vi "Add Unconfigured NICs.vi"(7 "ifconfig":string="# This file describes the network interfaces available on your system\n# and how to activate them. For more information, see interfaces(5).\n\n# The loopback network interface\nauto lo\niface lo inet loopback\n\n# The primary network interface\n#auto eth0\n#iface eth0 inet dhcp\n# Example to keep MAC address between reboots\n#hwaddress ether DE:AD:BE:EF:CA:FE\n\n# The secondary network interface\n#auto eth1\n#iface eth1 inet dhcp\n\n# WiFi Example\n#auto wlan0\n#iface wlan0 inet dhcp\n#    wpa-ssid \"essid\"\n#    wpa-psk  \"password\"\n\n# Ethernet/RNDIS gadget (g_ether)\n# Used by: /opt/scripts/boot/autoconfigure_usb0.sh\niface usb0 inet static\n    address 192.168.7.2\n    netmask 255.255.255.252\n    network 192.168.7.0\n    gateway 192.168.7.1e", 8 "Error In":errorcluster, 10 "All NIC Names":string[](array[string]), 11 "NIC Configs":T1[](array[typedef])) -> (0 "Error Out":errorcluster, 3 "NIC Configs":T1[](array[typedef]))   [LabVIEW 2020, in "LMH-LINX.lvlib"]
uses:
  LMH-LINX.lvlib
  NIC Info.ctl
  NIC Mode.ctl
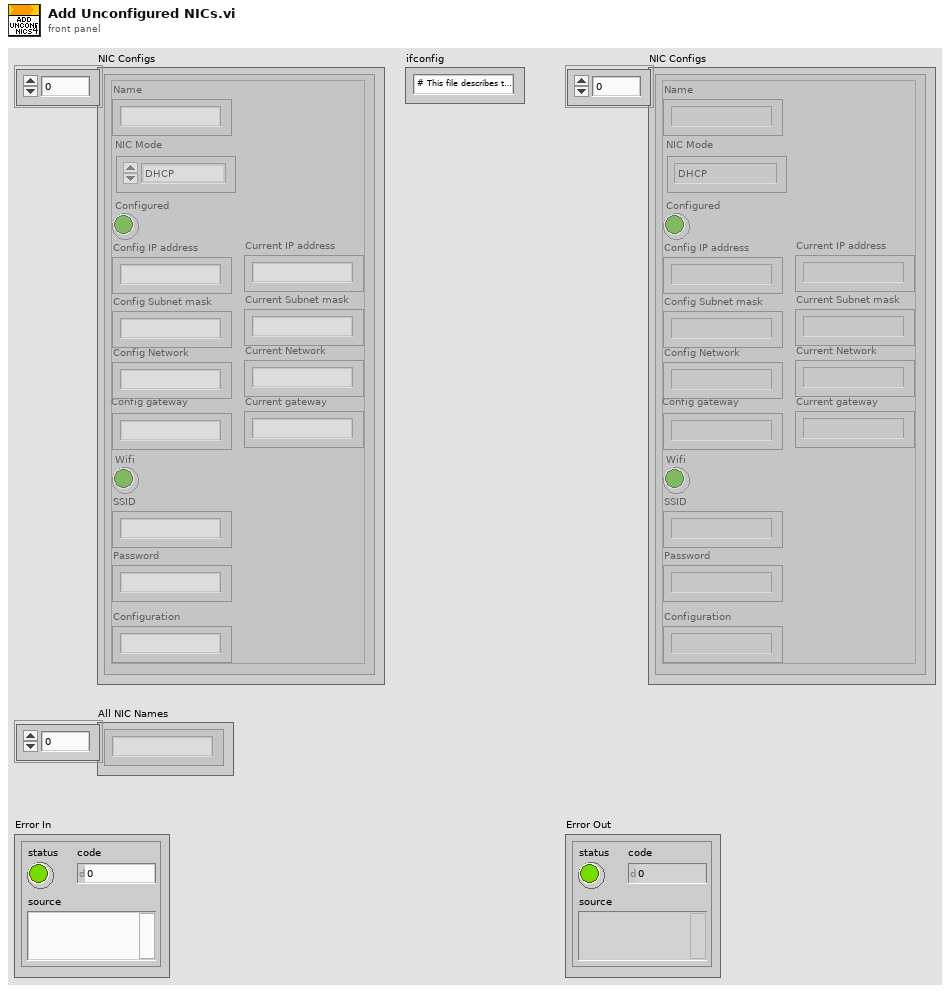
[diagram p1: front panel]
types:
  T1 = typedef "LMH-LINX.lvlib/NIC Info.ctl" = cluster{"Name":string, "NIC Mode":T2, "Configured":bool, "Config IP address":string, "Config Subnet mask":string, "Config Network":string, "Config gateway":string, "Wifi":bool, "SSID":string, "Password":string, "Configuration":string, "Current IP address":string, "Current Subnet mask":string, "Current gateway":string, "Current Network":string}
  T2 = typedef "LMH-LINX.lvlib/NIC Mode.ctl" = enum16{"DHCP", "Static", "Loopback"}
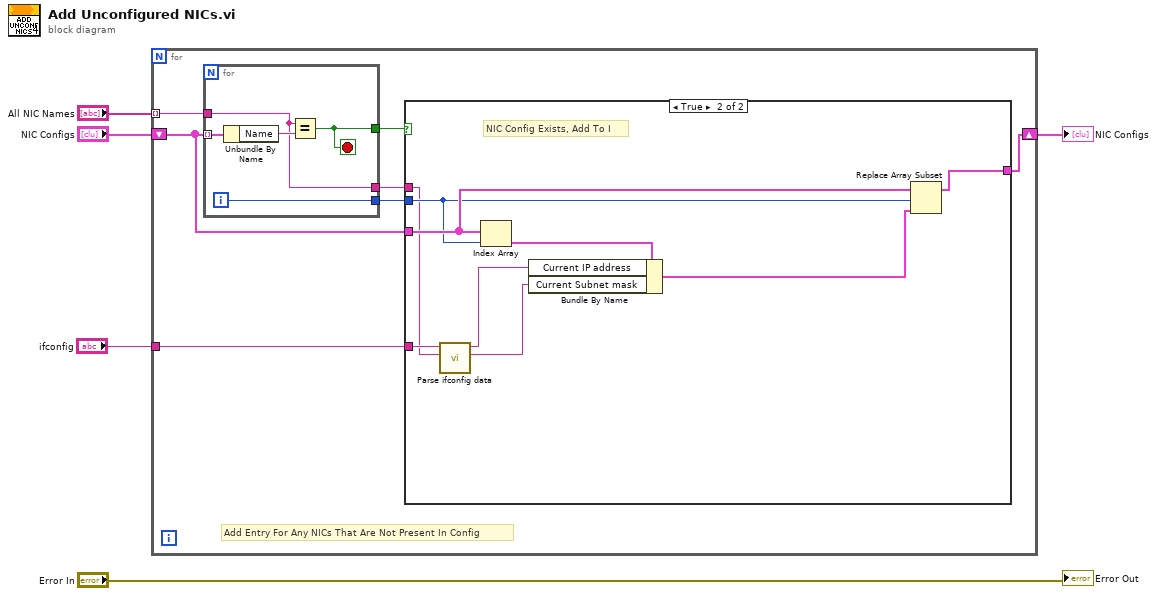
[diagram p0: block diagram]
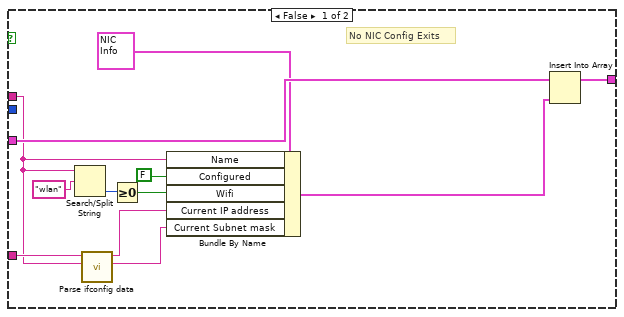
[diagram p2: hidden frame]
diagram:
  n1 = for {
    tunnel: "All NIC Names" -> [w7] mode=indexing
    shift-right: [w11] -> w5
    shift-left: "NIC Configs" -> [w9]
    tunnel: "ifconfig" -> [w8]
    # "Add Entry For Any NICs That Are Not Present In Config"
    n2 = for {
      tunnel: w9 -> [w36] mode=indexing
      tunnel: w7 -> [w35]
      tunnel: [w37] -> w12
      tunnel: [w35] -> w10
      tunnel: [w34] -> w6
      i -> [w34]
      stop <- w37 stop-if-true
      n3 = Unbundle By Name(w36) -> ("Name"=w38:string)
      n4 = Equal?(x=w35, y=w38) -> (x = y?=w37:bool)
    }
    n5 = case shown="True" w12 {
      tunnel: w9 -> [w24 w33]
      tunnel: [w23 w30] -> w11
      tunnel: w10 -> [w15 w25]
      tunnel: w8 -> [w19 w28]
      tunnel: w6 -> [_ w29]
      frame False {
        # "No NIC Config Exits"
        n6 = Search/Split String(string=w15, search string/char (-)="wlan") -> (offset of match=w18:i32)  [unwired: 1 in, 2 out]
        n7 = call "Parse ifconfig data.vi"("NIC Name"=w15, "ifconfig"=w19) -> ("Subnet mask"=w13:string, "IP Address"=w14:string)  [unwired: 8 in]
        n8 = Greater Or Equal To 0?(x=w18) -> (x >= 0?=w16:bool)
        n9 = Bundle By Name(cluster=T1 {"Name"="", "NIC Mode"=enum."DHCP", "Configured"=FALSE, "Config IP address"="", "Config Subnet mask"="", "Config Network"="", "Config gateway"="", "Wifi"=FALSE, "SSID"="", "Password"="", "Configuration"="", "Current IP address"="", "Current Subnet mask"="", "Current gateway"="", "Current Network"=""} ("NIC Info"), "Name"=w15, "Configured"=FALSE, "Wifi"=w16, "Current IP address"=w14, "Current Subnet mask"=w13) -> (w21:T1)
        n10 = Insert Into Array(array=w24, new element=w21) -> (w23:T1[])  [unwired: 1 in]
      }
      frame True {
        # "NIC Config Exists, Add To I"
        n11 = call "Parse ifconfig data.vi"("NIC Name"=w25, "ifconfig"=w28) -> ("Subnet mask"=w26:string, "IP Address"=w27:string)  [unwired: 8 in]
        n12 = Index Array(array=w33, index=w29) -> (element=w32:T1)
        n13 = Bundle By Name(cluster=w32, "Current IP address"=w27, "Current Subnet mask"=w26) -> (w31:T1)
        n14 = Replace Array Subset(array=w33, new element=w31, index=w29) -> (w30:T1[])
      }
    }
  }
  "NIC Configs" <- w5
  "Error Out" <- "Error In"
